vi "logger.vi"(11 "Message":string) -> ()   [LabVIEW 2023]
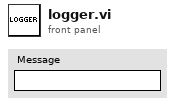
[diagram p1: front panel]
types:
  T1 = enum16{"open", "replace", "create", "open or create", "replace or create", "replace or create with confirmation"}
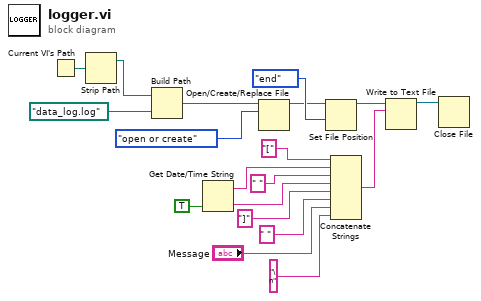
[diagram p0: block diagram]
diagram:
  n1 = Current VI's Path() -> (path=w19:path)
  n2 = Strip Path(path=w19) -> (stripped path=w18:path)  [unwired: 1 out]
  n3 = Build Path(base path=w18, name or relative path=path "data_log.log") -> (appended path=w16:path)
  n4 = Get Date/Time String(want seconds? (F)=TRUE) -> (date string=w9:string, time string=w6:string)  [unwired: 2 in]
  n5 = Open/Create/Replace File(file path (use dialog)=w16, operation (0:open)=T1."open or create") -> (refnum out=w12:refnum<file>)  [unwired: 4 in, 2 out]
  n6 = Set File Position(refnum=w12, from (0:start)=enum16{"start", "end", "current"}."end") -> (refnum out=w11:refnum<file>)  [unwired: 2 in, 1 out]
  n7 = Concatenate Strings("[" ("string"), w9, " " ("string"), w6, "]" ("string"), " " ("string"), "Message", "\n" ("string")) -> (w2:string)
  n8 = Write to Text File(file (use dialog)=w11, text=w2) -> (refnum out=w14:refnum<file>)  [unwired: 2 in, 2 out]
  n9 = Close File(refnum=w14) -> ()  [unwired: 1 in, 2 out]
